vi "addStreaming.vi"(7 "Streaming In":refnum<class "IStreaming.lvclass">, 8 "error in (no error)":errorcluster, 9 "Config in":refnum<class "IPropertyObject.lvclass">, 10 "ConnectionString in":string, 11 "IDevice in":refnum<class "IDevice.lvclass">) -> (0 "error out":errorcluster, 2 "Streaming out":refnum<class "IStreaming.lvclass">, 3 "IDevice out":refnum<class "IDevice.lvclass">)   [LabVIEW 2022 SP3, in "openDAQ.lvlib" / "IBaseObject.lvlib" / "IPropertyObject.lvlib" / "IComponent.lvlib" / "IFolder.lvlib" / "IDevice.lvlib" / "IDevice.lvclass"]
uses:
  <instrlib>/openDAQ/Public/Classes/IDevice/IDevice.lvclass
  <instrlib>/openDAQ/Public/Classes/IDevice/IDevice.lvclass/IDevice.ctl
  <instrlib>/openDAQ/Public/Classes/daqCoreTypes/IString/IString.lvclass
  <instrlib>/openDAQ/Public/Classes/IPropertyObject/IPropertyObject.lvclass
  <instrlib>/openDAQ/Public/Classes/IStreaming/IStreaming.lvclass
  <instrlib>/openDAQ/Binaries/Windows/x86/copendaq32.dll
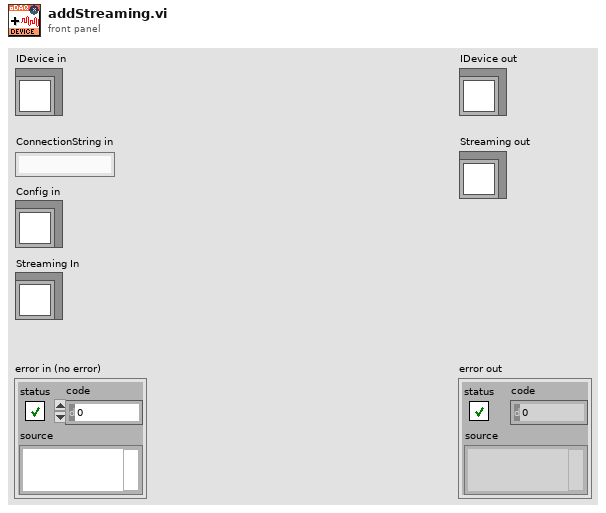
[diagram p1: front panel]
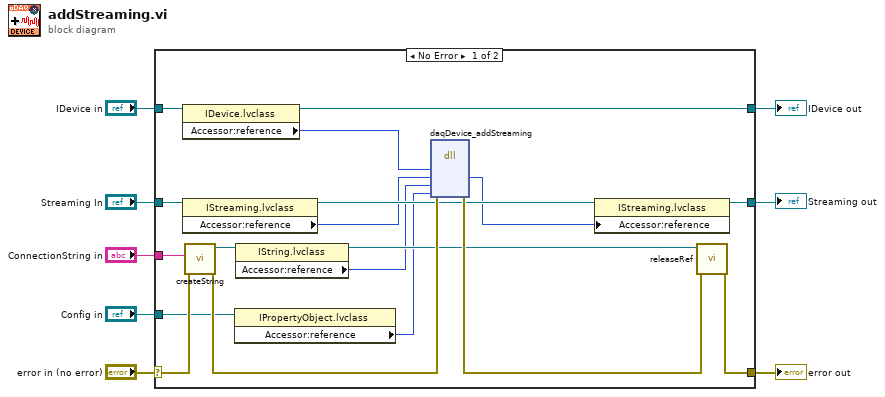
[diagram p0: block diagram]
diagram:
  n1 = case shown="No Error" "error in (no error)" {
    selector: "error in (no error)" -> [w16 w29]
    tunnel: [w13 w29] -> w7
    tunnel: [w22 w28] -> w5
    tunnel: "IDevice in" -> [w23 w28]
    tunnel: "Streaming In" -> [w21 w27]
    tunnel: [w20 w27] -> w3
    tunnel: "ConnectionString in" -> [w17 _]
    tunnel: "Config in" -> [w10 _]
    frame No Error {
      n2 = property class="IDevice.lvclass"(reference=w23) -> (reference out=w22:refnum<class "IDevice.lvclass">, "Accessor:reference"=w19:i64)  [unwired: 1 in, 1 out]
      n3 = property class="IStreaming.lvclass"(reference=w21) -> (reference out=w24:refnum<class "IStreaming.lvclass">, "Accessor:reference"=w18:i64)  [unwired: 1 in, 1 out]
      n4 = call <instrlib>:"createString.vi"("error in (no error)"=w16, "String"=w17) -> ("error out"=w26:errorcluster, "IString out"=w15:refnum<class "IString.lvclass">)  [unwired: 8 in]
      n5 = property class="IPropertyObject.lvclass"(reference=w10) -> ("Accessor:reference"=w9:i64)  [unwired: 1 in, 2 out]
      n6 = property class="IString.lvclass"(reference=w15) -> (reference out=w14:refnum<class "IString.lvclass">, "Accessor:reference"=w12:i64)  [unwired: 1 in, 1 out]
      n7 = dll-call lib="C:/Program Files (x86)/National Instruments/LabVIEW 2022/instr.lib/openDAQ/Binaries/Windows/x86/copendaq*.*" fn="daqDevice_addStreaming"(error in=w26, "device"=w19, "streaming"=w18, "connectionString"=w12, "config"=w9) -> (error out=w25:errorcluster, "streaming"=w11:i64)  [unwired: 6 in, 1 out]
      n8 = property class="IStreaming.lvclass"(reference=w24, "Accessor:reference"=w11) -> (reference out=w20:refnum<class "IStreaming.lvclass">)  [unwired: 1 in, 1 out]
      n9 = call-dynamic "releaseRef.vi"("error in (no error)"=w25, "IBaseObject in"=w14) -> ("error out"=w13:errorcluster)  [unwired: 9 in]
    }
    frame Error {
    }
  }
  "error out" <- w7
  "IDevice out" <- w5
  "Streaming out" <- w3
